vi "AG34980A_Fetch.vi"(0 "VISA resource name":refnum<visa-resource-name>, 7 "Numbers Only (T:On)":bool, 11 "error in (no error)":errorcluster, 12 "Byte Count (1024 bytes)":i32=1024) -> (4 "VISA resource name out":refnum<visa-resource-name>, 6 "Output Data (Numbers Only)":dbl[](array[numeric]) format="%.2e", 8 "Output Data":string[](array[string]), 15 "error out":errorcluster)   [LabVIEW 2022 SP3, in "DMM_Keysight_34980A.lvlib" / "DMM_Keysight_34980A.lvclass"]
doc: "This VI transfers readings from volatile memory to the instrument's output buffer where you can read them into your computer. The readings are not erased from memory when you read them. You can execute this VI multiple times to retrieve the same data in reading memory.\n\nWARNING: When \"Numbers Only\" is true, all data formatting must be disabled. If formatting is enabled, the results of this VI are undefined."
uses:
  DMM_Keysight_34980A.lvclass
  <vilib>/Utility/error.llb/Trim Whitespace One-Sided.vi
panel:
  # "WARNING: When \"Numbers Only\" is true, all data formatting must be disabled.  If formatting is enabled, the results of this VI are undefined."
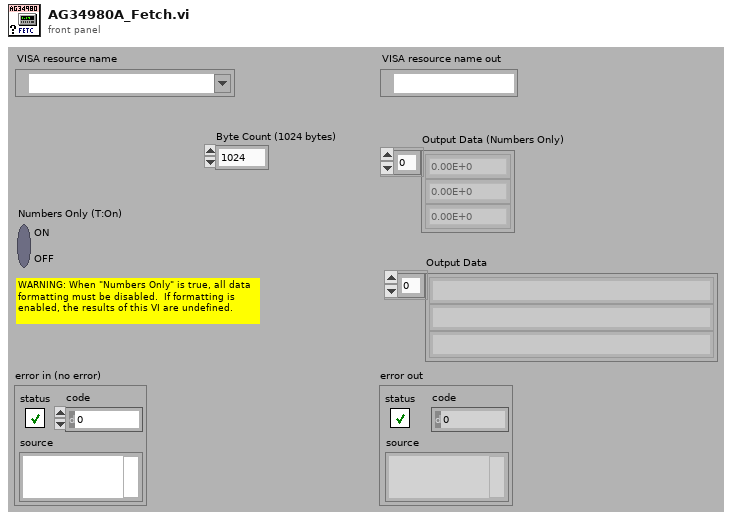
[diagram p1: front panel]
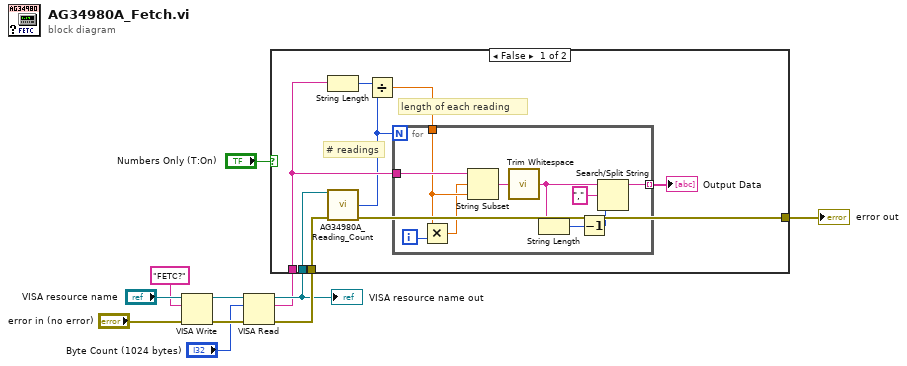
[diagram p0: block diagram]
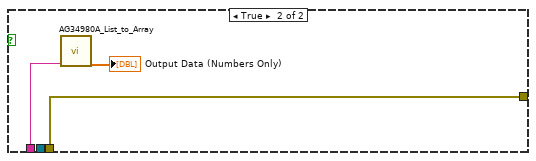
[diagram p2: hidden frame]
diagram:
  n1 = VISA Write(VISA resource name="VISA resource name", write buffer="FETC?", error in (no error)="error in (no error)") -> (VISA resource name out=w10:refnum<visa-resource-name>, error out=w9:errorcluster)  [unwired: 1 out]
  n2 = VISA Read(VISA resource name=w10, byte count="Byte Count (1024 bytes)", error in (no error)=w9) -> (VISA resource name out=w2:refnum<visa-resource-name>, read buffer=w1:string, error out=w11:errorcluster)  [unwired: 1 out]
  "VISA resource name out" <- w2
  n3 = case shown="False" "Numbers Only (T:On)" {
    tunnel: w1 -> [w16 w30]
    tunnel: w11 -> [w19 w31]
    tunnel: [w17 w31] -> w3
    tunnel: w2 -> [w12 _]
    frame False {
      # "length of each reading"
      # "# readings"
      n4 = String Length(string=w16) -> (length=w18:i32)
      n5 = call "AG34980A_Reading_Count.vi"("VISA resource name"=w12, "error in (no error)"=w19) -> ("Reading Count"=w13:u32, "error out"=w17:errorcluster)  [unwired: 11 in, 1 out]
      n6 = Divide(x=w18, y=w13) -> (x/y=w15:dbl)
      n7 = for {
        N: w13 -> [_]
        tunnel: w16 -> [w29]
        tunnel: w15 -> [w27]
        tunnel: [w21] -> w14 mode=indexing
        i -> [w28]
        n8 = Multiply(x=w27, y=w28) -> (x*y=w26:dbl)
        n9 = String Subset(string=w29, offset (0)=w26, length (rest)=w27) -> (substring=w25:string)
        n10 = call <vilib>:"Trim Whitespace.vi"("string"=w25) -> ("trimmed string"=w24:string)  [unwired: 1 in]
        n11 = String Length(string=w24) -> (length=w22:i32)
        n12 = Decrement(x=w22) -> (x-1=w20:i32)
        n13 = Search/Split String(string=w24, search string/char (-)=",", offset (0)=w20) -> (substring before match=w21:string)  [unwired: 2 out]
      }
      "Output Data" <- w14
    }
    frame True {
      n14 = call "AG34980A_List_to_Array.vi"("List"=w30) -> ("Output Number Array"=→"Output Data (Numbers Only)":dbl[])  [unwired: 5 in, 1 out]
    }
  }
  "error out" <- w3
